vi "ABC Start Position.vi"(4 "Start":cluster{"Steps":i32, "Rates":i32}, 6 "UART":refnum<vi>, 8 "ErrIn":errorcluster, 11 "ComPort":refnum<visa-resource-name>) -> (0 "ErrOut":errorcluster, 3 "LastPos":dbl)   [LabVIEW 2020]
uses:
  <userlib>/Amira UART/Public/TypeDefs/AUART StepDir.ctl
  <userlib>/Amira UART/Amira UART.lvclass
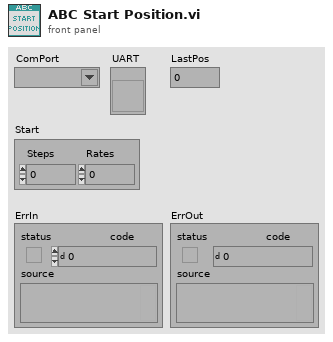
[diagram p1: front panel]
types:
  T1 = typedef "Amira UART.lvclass/AUART StepDir.ctl" = enum16{"", "compress", "decompress"}
  T2 = enum16{"", "100", "93.75", "87.5", "81.25", "75", "68.75", "62.5", "56.25", "50", "43.75", "37.5", "31.25", "25", "18.75", "12.5", "6.25"}
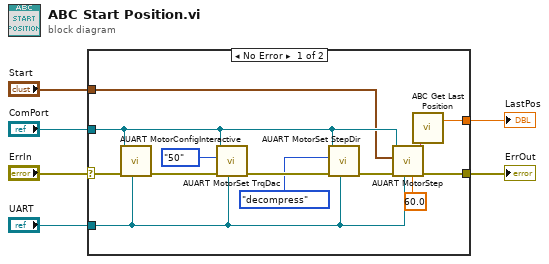
[diagram p0: block diagram]
diagram:
  n1 = case shown="No Error" "ErrIn" {
    selector: "ErrIn" -> [w10 w20]
    tunnel: "ComPort" -> [w15 _]
    tunnel: "UART" -> [w13 _]
    tunnel: "Start" -> [w12 _]
    tunnel: [w11 w20] -> w3
    tunnel: [w7 _] -> w1
    frame No Error {
      n2 = call <userlib>:"AUART MotorConfigInteractive.vi"("UART"=w13, "ErrIn"=w10, "Port"=w15) -> ("ErrOut"=w19:errorcluster)  [unwired: 8 in]
      n3 = call <userlib>:"AUART MotorSet TrqDac.vi"("UART"=w13, "ErrIn"=w19, "trq_dac"=T2."50", "Port"=w15) -> ("ErrOut"=w17:errorcluster)  [unwired: 7 in]
      n4 = call <userlib>:"AUART MotorSet StepDir.vi"("UART"=w13, "ErrIn"=w17, "step_dir"=AUART_StepDir."decompress", "Port"=w15) -> ("ErrOut"=w14:errorcluster)  [unwired: 7 in]
      n5 = call <userlib>:"AUART MotorStep.vi"("Timeout"=60.0, "UART"=w13, "ErrIn"=w14, "Vals"=w12, "Port"=w15) -> ("ErrOut"=w11:errorcluster, "Response"=w8:string)  [unwired: 5 in]
      n6 = call "ABC Get Last Position.vi"("Response"=w8) -> ("Position"=w7:dbl)  [unwired: 1 in]
    }
    frame Error {
    }
  }
  "ErrOut" <- w3
  "LastPos" <- w1
